vi "EuniceF_Project5_Labview.vi"() -> ()   [LabVIEW 2025]
panel:
  out "HEATING":bool
  in  "STOP":bool
  out "COOLING":bool
  out "Thermometer":dbl(slide) scale=0.0..100.0
  out "Vscc,V":dbl(slide) scale=0.0..10.0
  out "AtoD":i16
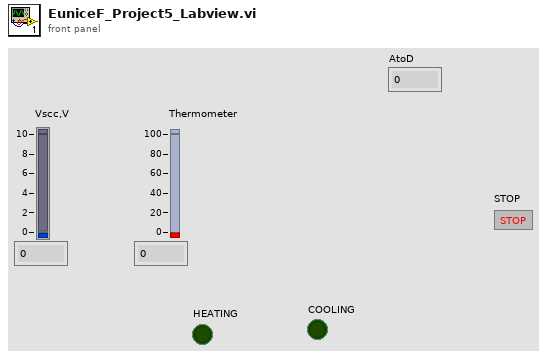
[diagram p1: front panel]
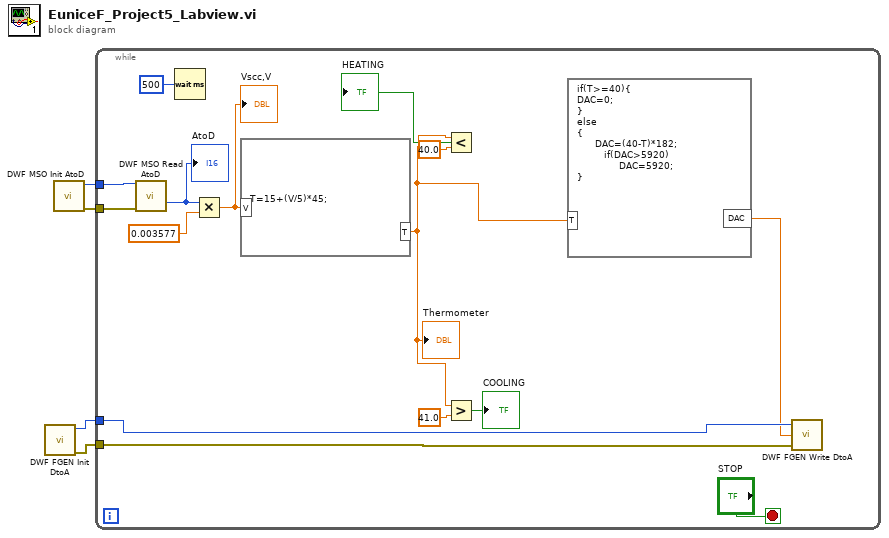
[diagram p0: block diagram]
diagram:
  n1 = call "DWF FGEN Init DtoA.vi"() -> ("Error Out"=w1:errorcluster, "Instrument Handle Out"=w2:u32)  [unwired: 10 in]
  n2 = call "DWF MSO Init AtoD.vi"() -> ("Error Out"=w3:errorcluster, "Instrument Handle Out"=w4:i32)  [unwired: 10 in]
  n3 = while {
    tunnel: w4 -> [w19]
    tunnel: w3 -> [w18]
    tunnel: w2 -> [w9]
    tunnel: w1 -> [w8]
    stop <- "STOP" stop-if-true
    n4 = call "DWF MSO Read AtoD.vi"("Instrument Handle In AtoD"=w19, "Error In"=w18) -> ("AtoD"=w17:i16)  [unwired: 12 in, 1 out]
    "AtoD" <- w17
    n5 = Wait (ms)(milliseconds to wait=u32 500) -> ()  [unwired: 1 out]
    n6 = Multiply(x=w17, y=0.003577) -> (x*y=w15:dbl)
    "Vscc,V" <- w15
    n7 = formula code="T=15+(V/5)*45;"("V"=w15) -> ("T"=w7:dbl)
    "Thermometer" <- w7
    n8 = Less?(x=w7, y=40.0) -> (x < y?=→"HEATING":bool)
    n9 = Greater?(x=w7, y=41.0) -> (0:→"COOLING":bool)
    n10 = formula code="if(T>=40){\nDAC=0;\n}\nelse\n{\n      DAC=(40-T)*182;\n         if(DAC>5920)\n              DAC=5920;\n}"("T"=w7) -> ("DAC"=w5:dbl)
    n11 = call "DWF FGEN Write DtoA.vi"("Error In"=w8, "Raw Data"=w5, "Instrument Handle In"=w9) -> ()  [unwired: 1 in, 2 out]
  }
